vi "Release Session.vi"(6 "force destroy? (F)":bool, 8 "error in":errorcluster, 11 "Session Handle":T1) -> (0 "error out":errorcluster, 3 "file path":path)   [LabVIEW 2014, in "Config Data.lvclass"]
doc: "Release the configuration session for the given reference. If this is the last reference to return, then the config data file will be closed and the file path for the configuration file will be returned."
uses:
  Config Data.lvclass
  <userlib>/_Session Fwk/Session - Root.lvclass
  <vilib>/Utility/config.llb/NI_LVConfig.lvlib
  Config Session.ctl
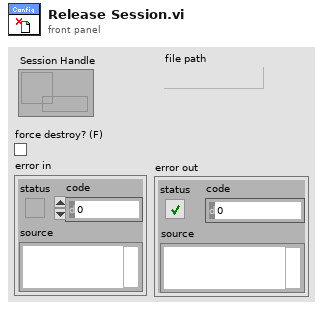
[diagram p1: front panel]
types:
  T1 = typedef "Config Data.lvclass/Config Session.ctl" = refnum<data-value>
  T2 = typedef "NI_LVConfig.lvlib/Config Data RefNum.ctl" = refnum<k1>
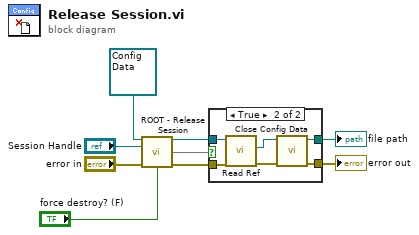
[diagram p0: block diagram]
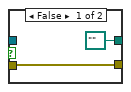
[diagram p2: hidden frame]
diagram:
  n1 = call <userlib>:"ROOT - Release Session.vi"("OBJ - Session in"=refnum<class "Config Data.lvclass"> refnum ("Config Data"), "Session Handle in"="Session Handle", "error in (no error)"="error in", "force destroy? (F)"="force destroy? (F)") -> ("OBJ - Session out"=w5:refnum<class "Config Data.lvclass">, 8:w6, "error out"=w4:errorcluster)  [unwired: 9 in]
  n2 = case shown="True" w6 {
    tunnel: w5 -> [_ w17]
    tunnel: w4 -> [w10 w16]
    tunnel: [w10 w13] -> w2
    tunnel: [path "" ("file path") w12] -> w1
    frame False {
    }
    frame True {
      n3 = call "Read Ref.vi"("error in"=w16, "Config Data in"=w17) -> ("error out"=w14:errorcluster, "config data"=w15:T2)  [unwired: 7 in, 1 out]
      n4 = call <vilib>:"Close Config Data.vi"("error in (no error)"=w14, "refnum"=w15) -> ("error out"=w13:errorcluster, "file path"=w12:path)  [unwired: 8 in]
    }
  }
  "error out" <- w2
  "file path" <- w1
